vi "Create SFOAE Test Data.vi"() -> ()   [LabVIEW 2015]
uses:
  Typedefs/SFOAE-Stimulus Parameters.ctl
  Typedefs/SFOAE-Sweep Params.ctl
  Typedefs/SFOAE-Data Processing.ctl
  Utility VIs/Math VIs/LinSpace (start-stop-step).vi
  Utility VIs/Math VIs/Linear to dB (scalar).vi
  <vilib>/Analysis/NI_AALBase.lvlib
panel:
  out "Phase":cluster{"Array":dbl[], "Array":dbl[]}[](graph)
  out "Mag":cluster{"Array":dbl[], "Array":dbl[]}[](graph)
  out "Stim":cluster{"Array":dbl[], "Array":dbl[]}[](graph) caption="Raw"
  out "SeqStep":i32
  out "Nacq":i32
  out "frame pts":i32=50000
  out "data proc":T1={"dt (ms)"=0.01, "TrialLen"=144000, "PT"=[], "CurPos"=0, "Sum"=[], "Navg"=[], "Nacq"=4, "RawPath"=path "", "DataPath"=path "", "NumToAcq"=4, "OAE"=array[48000 elements], "CurTrial"=array[144000 elements], "StimLen"=48000, "SFOAE"=[], "SeqStep"=0, "updated"=TRUE, "SeqVals"=[], "df (kHz)"=0.0020833333333333333, "MagRef"=refnum, "LastOAE"=[], "OAE Diff Sum"=[], "Noise Floor"=[], "SpecFactor"=0.0, "Offset"=0, "Nfft"=0, "PhsRef"=refnum}
  out "Avg":cluster{"Array":dbl[], "Array":dbl[]}[](graph) caption="Raw"
  out "Raw":cluster{"Array":dbl[], "Array":dbl[]}(graph)
  in  "Frame size (s)":dbl=0.5
  in  "Cal Folder":path=path "C:/Experiment VIs/Cochlear Function Test Suite/LV Source/SFOAE VIs/Test VIs"
  in  "Fs (Hz)":dbl=100000.0
  in  "SFOAE Stim":T2={"Ear"=enum."Right", "Sweep"={"Type"=enum."Linear", "Fmin (kHz)"=4.0, "Fmax (kHz)"=44.0, "Rate"=5.0, "Ramp (ms)"=20.0, "Drain (ms)"=20.0}, "Suppressor"={"Delta"=50.0, "Ratio"=0.0, "Use ratio"=FALSE}, "Concurrent"={"Nsweeps"=4, "Overlap"=0.0}, "Ls (dB SPL)"=-23.0, "Lp (dB SPL)"={"Min"=-23.0, "Max"=-23.0, "Step"=10.0}}
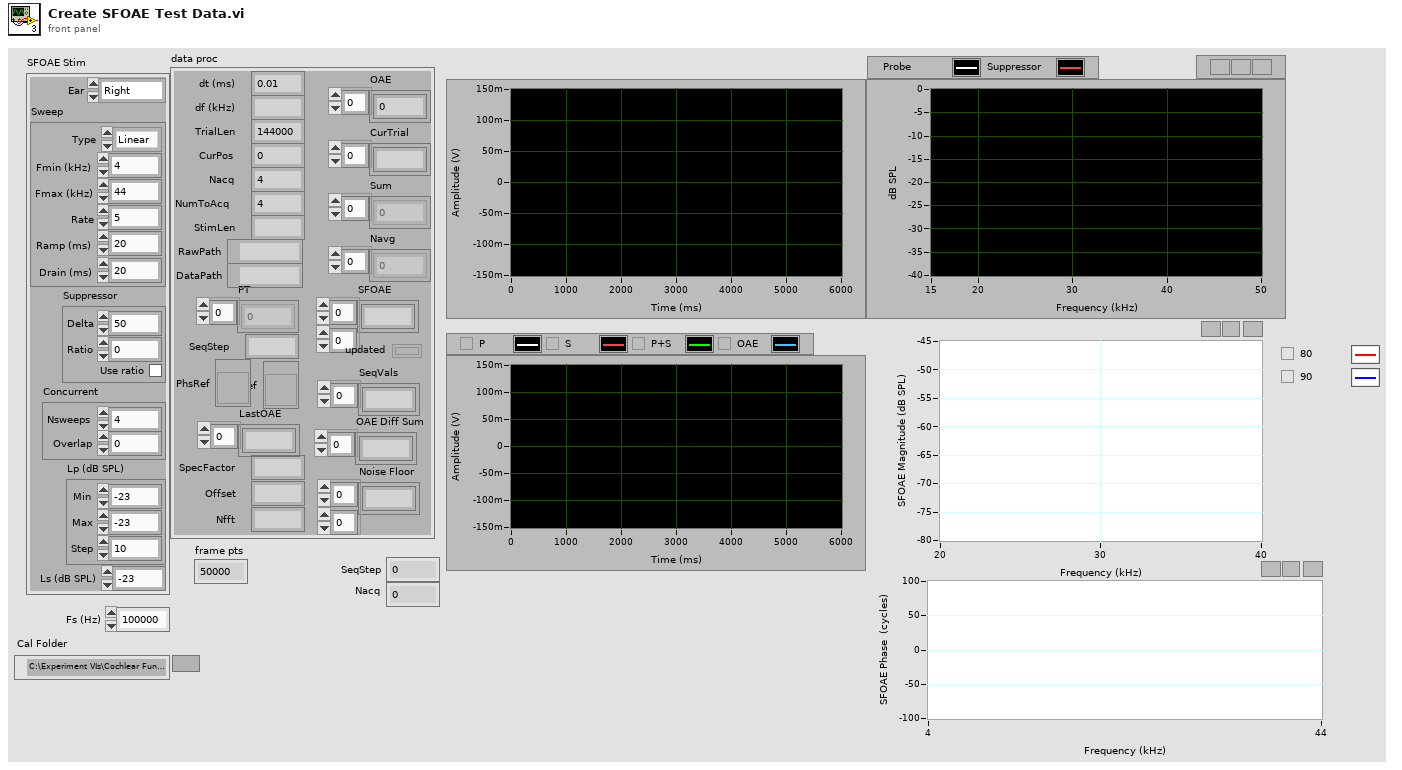
[diagram p1: front panel]
types:
  T1 = typedef "SFOAE-Data Processing.ctl" = cluster{"dt (ms)":dbl, "TrialLen":i32, "PT":cdb[], "CurPos":i32, "Sum":dbl[], "Navg":dbl[], "Nacq":i32, "RawPath":path, "DataPath":path, "NumToAcq":i32, "OAE":dbl[], "CurTrial":dbl[], "StimLen":i32, "SFOAE":cdb[][], "SeqStep":i32, "updated":bool, "SeqVals":dbl[], "df (kHz)":dbl, "MagRef":refnum<vi>, "LastOAE":dbl[], "OAE Diff Sum":dbl[], "Noise Floor":cdb[][], "SpecFactor":dbl, "Offset":i32, "Nfft":i32, "PhsRef":refnum<vi>}
  T2 = typedef "SFOAE-Stimulus Parameters.ctl" = cluster{"Ear":enum16{"Right", "Left"}, "Sweep":T3, "Suppressor":cluster{"Delta":dbl, "Ratio":dbl, "Use ratio":bool}, "Concurrent":cluster{"Nsweeps":i32, "Overlap":dbl}, "Ls (dB SPL)":dbl, "Lp (dB SPL)":cluster{"Min":dbl, "Max":dbl, "Step":dbl}}
  T3 = typedef "SFOAE-Sweep Params.ctl" = cluster{"Type":enum16{"Linear", "Log"}, "Fmin (kHz)":dbl, "Fmax (kHz)":dbl, "Rate":dbl, "Ramp (ms)":dbl, "Drain (ms)":dbl}
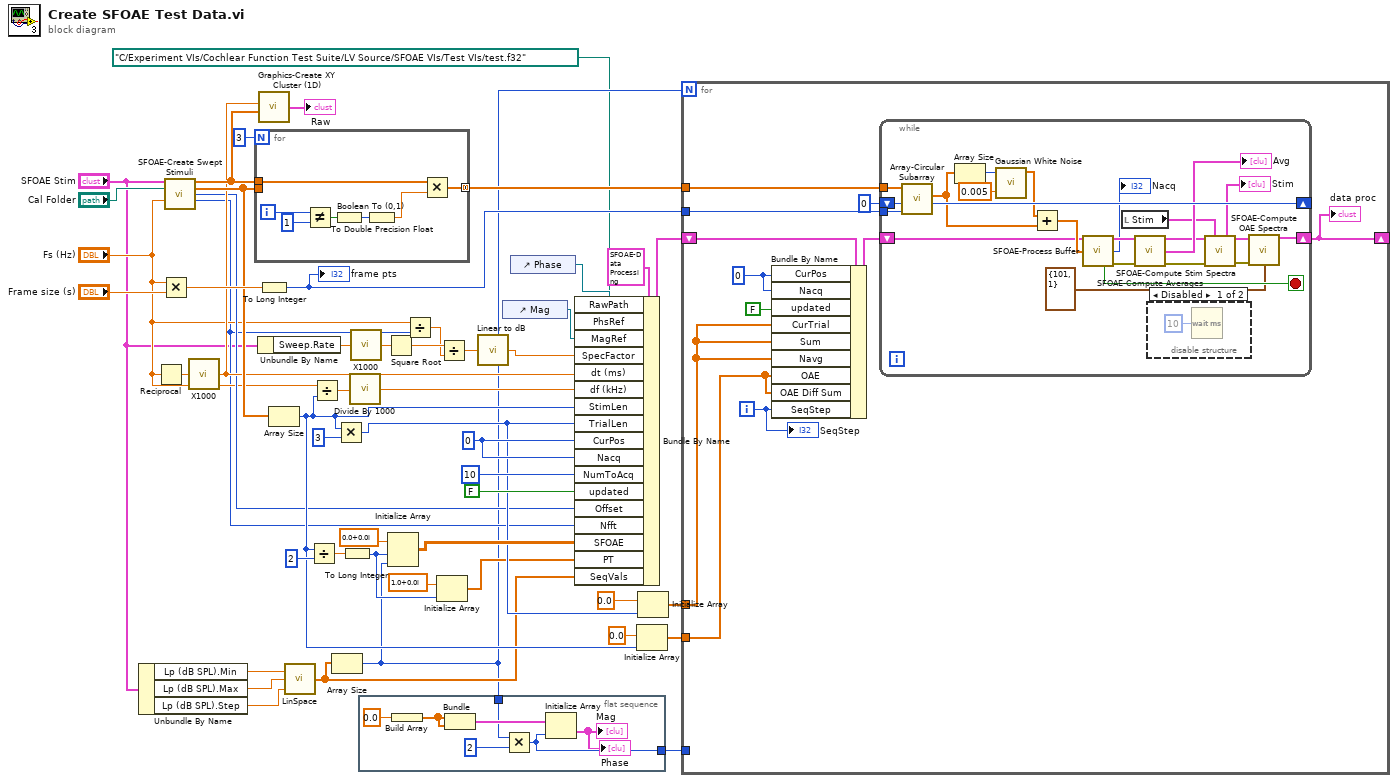
[diagram p0: block diagram]
diagram:
  w38 = 0 ("CurPos")
  n1 = Unbundle By Name("SFOAE Stim") -> ("Lp (dB SPL).Min"=w19:dbl, "Lp (dB SPL).Max"=w18:dbl, "Lp (dB SPL).Step"=w17:dbl)
  n2 = Reciprocal(x="Fs (Hz)") -> (1/x=w43:dbl)
  n3 = Multiply(x="Fs (Hz)", y="Frame size (s)") -> (x*y=w47:dbl)
  n4 = call "SFOAE-Create Swept Stimuli.vi"("SFOAE Stim"="SFOAE Stim", "Data Folder"="Cal Folder", "Fs (Hz)"="Fs (Hz)") -> ("probe"=w23:dbl[], "suppressor"=w42:dbl[], "offset"=w15:i32, "nfft"=w8:i32)  [unwired: 8 in, 1 out]
  n5 = call "X1000.vi"("X"=w43) -> ("X/1000"=w22:dbl)
  n6 = for {
    N: 3 -> [_]
    tunnel: w23 -> [w54]
    tunnel: w42 -> [_]
    tunnel: [w52] -> w49 mode=concatenating
    i -> [w58]
    n7 = Not Equal?(x=w58, y=1) -> (x != y?=w56:bool)
    n8 = Boolean To (0,1)(Boolean=w56) -> (0, 1=w55:i16)
    n9 = To Double Precision Float(number=w55) -> (double precision float=w53:dbl)
    n10 = Multiply(x=w54, y=w53) -> (x*y=w52:dbl[])
  }
  n11 = Unbundle By Name("SFOAE Stim") -> ("Sweep.Rate"=w10:dbl)
  n12 = call "Graphics-Create XY Cluster (1D).vi"("Array"=w23, "dx"=w22) -> ("XY cluster"=→"Raw":cluster{"Array":dbl[], "Array":dbl[]})  [unwired: 2 in]
  n13 = To Long Integer(number=w47) -> (32bit integer=w46:i32)
  "frame pts" <- w46
  n14 = Array Size(array=w42) -> (size(s)=w28:i32)
  n15 = call-poly "LinSpace.vi"("Step"=w17, "Stop"=w18, "Start"=w19) -> ("Array"=w16:dbl[])  [unwired: 1 in, 1 out]
  n16 = Divide(x=w28, y=2) -> (x/y=w34:dbl)
  n17 = Divide(x="Fs (Hz)", y=w28) -> (x/y=w41:dbl)
  n18 = Array Size(array=w16) -> (size(s)=w6:i32)
  n19 = Multiply(x=w28, y=3) -> (x*y=w29:i32)
  n20 = To Long Integer(number=w34) -> (32bit integer=w26:i32)
  n21 = call "Divide By 1000.vi"("X"=w41) -> ("X/1000"=w40:dbl)
  n22 = call "X1000.vi"("X"=w10) -> ("X/1000"=w11:dbl)
  n23 = flat-sequence {
    tunnel: w6 -> [w61]
    tunnel: [w60] -> w5
    frame #0 {
      n24 = Build Array(0.0) -> (w62:dbl[])
      n25 = Bundle(w62, w62) -> (w65:cluster{dbl[], dbl[]})  [unwired: 1 in]
      n26 = Multiply(x=w61, y=2) -> (x*y=w60:i32)
      n27 = Initialize Array(w65, w60) -> (→"Mag" →"Phase":cluster{dbl[], dbl[]}[])
    }
  }
  n28 = Square Root(x=w11) -> (sqrt(x)=w14:dbl)
  n29 = Initialize Array(cdb 0.0+0.0i ("element"), w26, w6) -> (w32:cdb[][])
  n30 = Divide(x="Fs (Hz)", y=w8) -> (x/y=w13:dbl)
  n31 = Initialize Array(cdb 1.0+0.0i ("element"), w26) -> (w25:cdb[])
  n32 = Divide(x=w14, y=w13) -> (x/y=w12:dbl)
  n33 = call-poly "Linear to dB.vi"("Linear"=w12) -> ("dB"=w1:dbl)
  n34 = control-ref of="Mag"() -> (w7:refnum<vi>)
  n35 = control-ref of="Phase"() -> (w3:refnum<vi>)
  n36 = Bundle By Name(cluster=T1 {"dt (ms)"=0.0, "TrialLen"=0, "PT"=[], "CurPos"=0, "Sum"=[], "Navg"=[], "Nacq"=0, "RawPath"=path "", "DataPath"=path "", "NumToAcq"=0, "OAE"=[], "CurTrial"=[], "StimLen"=0, "SFOAE"=[], "SeqStep"=0, "updated"=FALSE, "SeqVals"=[], "df (kHz)"=0.0, "MagRef"=refnum, "LastOAE"=[], "OAE Diff Sum"=[], "Noise Floor"=[], "SpecFactor"=0.0, "Offset"=0, "Nfft"=0, "PhsRef"=refnum} ("DataProc In"), "RawPath"=path "C:/Experiment VIs/Cochlear Function Test Suite/LV Source/SFOAE VIs/Test VIs/test.f32", "PhsRef"=w3, "MagRef"=w7, "SpecFactor"=w1, "dt (ms)"=w22, "df (kHz)"=w40, "StimLen"=w28, "TrialLen"=w29, "CurPos"=w38, "Nacq"=w38, "NumToAcq"=10, "updated"=FALSE, "Offset"=w15, "Nfft"=w8, "SFOAE"=w32, "PT"=w25, "SeqVals"=w16) -> (w44:T1)
  n37 = Initialize Array(0.0 ("element"), w28) -> (w20:dbl[])
  n38 = Initialize Array(0.0 ("element"), w29) -> (w21:dbl[])
  n39 = for {
    N: w6 -> [_]
    tunnel: w49 -> [w76]
    tunnel: w46 -> [w75]
    shift-right: [w73] -> _
    shift-left: w44 -> [w72]
    tunnel: w21 -> [w67]
    tunnel: w20 -> [w66]
    tunnel: w5 -> [_]
    i -> [w68]
    w70 = 0 ("CurPos")
    n40 = Bundle By Name(cluster=w72, "CurPos"=w70, "Nacq"=w70, "updated"=FALSE, "CurTrial"=w67, "Sum"=w67, "Navg"=w67, "OAE"=w66, "OAE Diff Sum"=w66, "SeqStep"=w68) -> (w71:T1)
    n41 = while {
      tunnel: w76 -> [w99]
      tunnel: w75 -> [w98]
      shift-right: [w97] -> _
      shift-left: 0 ("Offset (out)") -> [w96]
      shift-right: [w81] -> w73
      shift-left: w71 -> [w77]
      stop <- w93 stop-if-true
      n42 = call "Array-Circular Subarray.vi"("Npts"=w98, "Offset (in)"=w96, "Array"=w99) -> ("Offset (out)"=w97:i32, "Subarray"=w78:dbl[])  [unwired: 7 in]
      n43 = Array Size(array=w78) -> (size(s)=w85:i32)
      n44 = call <vilib>:"Gaussian White Noise.vi"("standard deviation"=0.005, "samples"=w85) -> ("Gaussian noise pattern"=w84:dbl[])  [unwired: 8 in, 1 out]
      n45 = Add(x=w84, y=w78) -> (x+y=w86:dbl[])
      n46 = call "SFOAE-Process Buffer.vi"("DataProc In"=w77, "Buffer"=w86) -> ("DataProc Out"=w94:T1, "Nacq"=→"Nacq":i32, "Finished"=w93:bool, "error out"=w95:errorcluster)  [unwired: 10 in]
      n47 = local read "Stim"() -> (w87:cluster{"Array":dbl[], "Array":dbl[]}[])
      n48 = call "SFOAE-Compute Averages.vi"("DataProc In"=w94, "error in (no error)"=w95) -> ("DataProc Out"=w90:T1, "Graph Array"=→"Avg":cluster{"Array":dbl[], "Array":dbl[]}[], "error out"=w89:errorcluster)  [unwired: 11 in]
      n49 = disable-structure shown="Disabled" {
        frame Disabled {
          n50 = Wait (ms)(milliseconds to wait=u32 10) -> ()  [unwired: 1 out]
        }
        frame Enabled {
        }
      }
      n51 = call "SFOAE-Compute Stim Spectra.vi"("DataProc In"=w90, "MagSpect In"=w87, "error in (no error)"=w89) -> ("MagSpect"=→"Stim":cluster{"Array":dbl[], "Array":dbl[]}[], "DataProc Out"=w82:T1, "error out"=w80:errorcluster)  [unwired: 10 in]
      n52 = call "SFOAE-Compute OAE Spectra.vi"("DataProc In"=w82, "error in (no error)"=w80, "Smoothing"=cluster{"Length":i32, "Iterations":i32} {"Length"=101, "Iterations"=1}) -> ("DataProc Out"=w81:T1)  [unwired: 11 in, 1 out]
    }
    "data proc" <- w73
    "SeqStep" <- w68
  }
